vi "2DNonlinear Lev-Mar Fit.vi"(5 "Standard Deviation":dbl[](array[numeric]) format="%.2f", 7 "Function":refnum<vi>, 8 "max iteration":i32=200, 9 "Initial Guess Coefficients":dbl[](array[numeric]) format="%.2f", 10 "Y":dbl[](array[numeric]) format="%.2f", 11 "X":dbl[](array[numeric]) format="%.2f") -> (0 "error":i32, 1 "mse":dbl format="%.4e", 2 "Best Fit":dbl[](array[numeric]) format="%.2f", 3 "Best Fit Coefficients":dbl[](array[numeric]) format="%.2f", 4 "Covariance":dbl[][](array[numeric]) format="%.2f")   [LabVIEW 2016]
doc: "NonLinear Lev-Mar Fit:\n==================\n\nThis VI uses the Levenberg-Marquardt algorithm to determine the least squares set of coefficients that best fit the set of input data points(X,Y) as expressed by a nonlinear function y=f(x,a) where a is the set of coefficients. This VI also gives the best fit curve y=f(x.a). \n\nThe user needs to open a sub-VI \"Target Fnc & Deriv NonLin\" and inputs his/her nonlinear function f(x,a) in the Formula Node. If the user choose formula caculation for derivative method, he/she needs to input the partial deriative of f(x,a) with respect to a as well. \n\nInputs:\nX: experiment data points.\nY: experiment data points.\nStandard Deviation: standard deviation of each experiment data.If you don't have knowledge about this parameter, just leave it empty.\nInitial Guess Coefficients: Your guessed coefficients. If this is too far from the appropriate coefficients, the VI maybe will fail to return the appropriate coeficients and best fit curve.\nmax iteration: max iteration the algrothim will try. If it can not converge when it reaches the max iteration. The VI will return an error.\nderivative: There are two ways to caculate the partial derivative of f(x,a) with respect to coefficients a. If you choose nemerical caculation, the VI will use numerical method to caculate them internally. If you choose formula caculation, you need to input the derivative formula in the subvi Target Fnc & Deriv NonLin. formula caculation is more precise than numerical caculation.\n\nOutputs:\nBest Guess Coefficients: the least squares coefficients.\nBest Fit: the best fit curve f(x,a).\nCovariance: covariance matrix of Best Guess Coefficients.\nmse: mse=1/n*sum[(y(i)-f(x(i),a))/std(i)]^2)\n (std: Standard Deviation)"
uses:
  <vilib>/Analysis/baseanly.llb/Real Inverse Matrix.vi
  <vilib>/Analysis/NI_AALPro.lvlib
  <vilib>/Analysis/NI_AALBase.lvlib
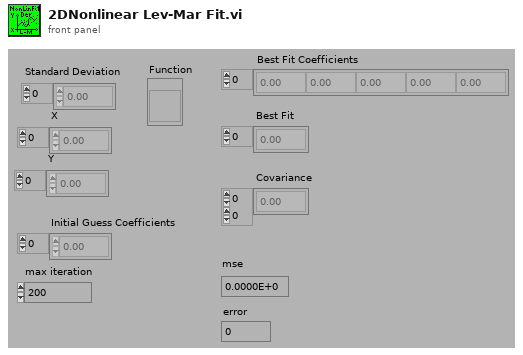
[diagram p1: front panel]
types:
  T1 = typedef "NI_Matrix.lvlib/RealMatrix.ctl" = dbl[][]
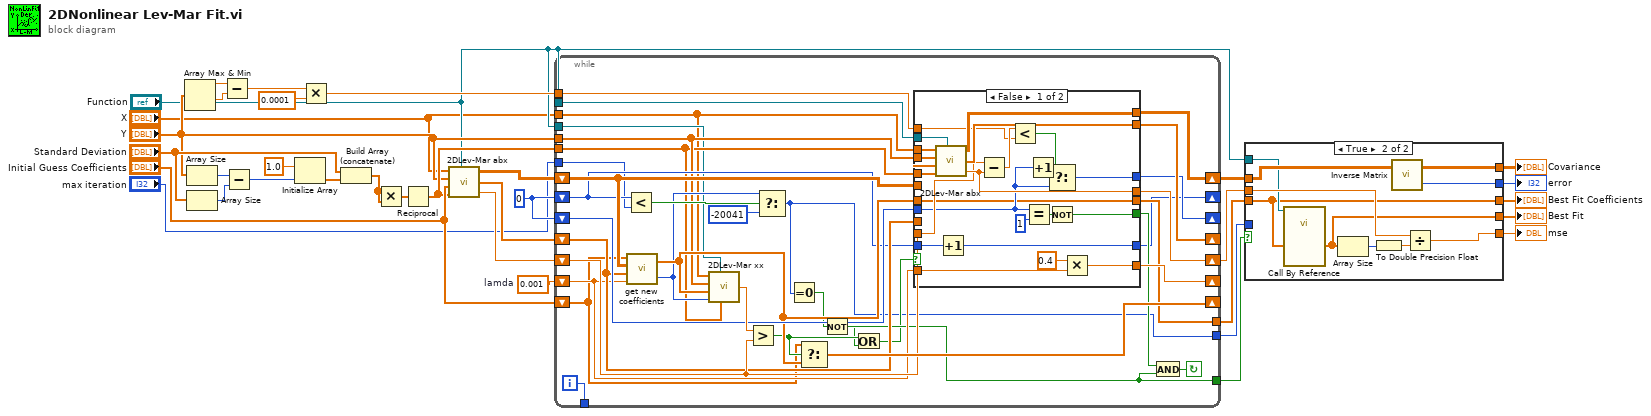
[diagram p0: block diagram]
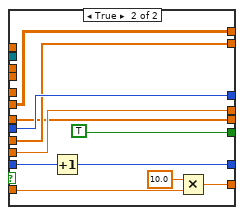
[diagram p2: hidden frame]
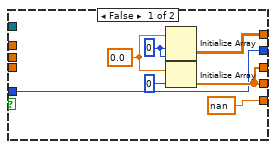
[diagram p3: hidden frame]
diagram:
  w25 = 0
  w33 = 0.001  # lamda
  n1 = Array Max & Min(array="Y") -> (max value=w7:dbl, min value=w6:dbl)  [unwired: 2 out]
  n2 = Array Size(array="Y") -> (size(s)=w13:i32)
  n3 = Array Size(array="Standard Deviation") -> (size(s)=w14:i32)
  n4 = Subtract(x=w7, y=w6) -> (x-y=w5:dbl)
  n5 = Subtract(x=w13, y=w14) -> (x-y=w15:i32)
  n6 = Initialize Array(1.0, w15) -> (w16:dbl[])
  n7 = Multiply(x=w5, y=0.0001) -> (x*y=w4:dbl)
  n8 = Build Array (concatenate)("Standard Deviation", w16) -> (w9:dbl[])
  n9 = Multiply(x=w9, y=w9) -> (x*y=w11:dbl[])
  n10 = Reciprocal(x=w11) -> (1/x=w10:dbl[])
  n11 = call "2DLev-Mar abx.vi"("X"="X", "Function"="Function", "Y"="Y", "Coefficients"="Initial Guess Coefficients", "W"=w10) -> ("Alpha"=w34:dbl[][], "Beta"=w32:dbl[], "chiSqr"=w31:dbl)  [unwired: 1 in]
  n12 = while {
    tunnel: "Function" -> [w37]
    tunnel: "Function" -> [w38]
    shift-right: [w68] -> _
    shift-left: w33 -> [w57]
    shift-right: [w67] -> _
    shift-left: "Initial Guess Coefficients" -> [w40]
    shift-right: [w66] -> w18
    shift-left: w34 -> [w65]
    shift-right: [w64] -> _
    shift-left: w32 -> [w59]
    shift-right: [w63] -> w30
    shift-left: w31 -> [w62]
    shift-right: [w60] -> _
    shift-left: w25 -> [w61]
    tunnel: [w56] -> w29
    tunnel: [w53] -> w26
    tunnel: w4 -> [w52]
    shift-right: [w48] -> _
    shift-left: w25 -> [w47]
    tunnel: "max iteration" -> [w43]
    tunnel: [w42] -> w19
    tunnel: "Y" -> [w41]
    tunnel: w10 -> [w39]
    tunnel: "X" -> [w36]
    tunnel: [w35] -> _
    i -> [w35]
    stop <- w55 continue-if-true
    n13 = Less?(x=w47, y=w43) -> (x < y?=w46:bool)
    n14 = call <vilib>:"get new coefficients.vi"("lamda"=w57, "Beta"=w59, "Alpha"=w65, "Coefficients"=w40) -> ("error"=w44:i32, "New Coefficients"=w58:dbl[])
    n15 = call "2DLev-Mar xx.vi"("W"=w39, "Function"=w37, "error"=w44, "Coefficients"=w58, "Y"=w41, "X"=w36) -> ("chiSqr"=w69:dbl)
    n16 = Greater?(x=w69, y=w62) -> (0:w50:bool)
    n17 = Select(t=w44, s=w46, f=-20041) -> (s? t:f=w42:i32)
    n18 = Equal To 0?(x=w42) -> (x = 0?=w53:bool)
    n19 = Select(t=w40, s=w50, f=w58) -> (s? t:f=w67:dbl[])
    n20 = Not(x=w53) -> (.not. x?=w49:bool)
    n21 = Or(x=w50, y=w49) -> (x .or. y?=w51:bool)
    n22 = case shown="False" w51 {
      tunnel: w57 -> [w91 w102]
      tunnel: [w90 w101] -> w68
      tunnel: [w89 w100] -> w66
      tunnel: w65 -> [_ w100]
      tunnel: [w88 w96] -> w64
      tunnel: [w87 w99] -> w63
      tunnel: w62 -> [w86 w99]
      tunnel: w61 -> [w81 w98]
      tunnel: [w82 w98] -> w60
      tunnel: [w78 TRUE] -> w54
      tunnel: w58 -> [w75 w95]
      tunnel: w59 -> [_ w96]
      tunnel: [w75 w95] -> w56
      tunnel: w52 -> [w77 _]
      tunnel: [w74 w94] -> w48
      tunnel: w47 -> [w76 w93]
      tunnel: w41 -> [w73 _]
      tunnel: w39 -> [w72 _]
      tunnel: w38 -> [w71 _]
      tunnel: w36 -> [w70 _]
      frame False {
        n23 = call "2DLev-Mar abx.vi"("X"=w70, "Function"=w71, "Y"=w73, "Coefficients"=w75, "W"=w72) -> ("Alpha"=w89:dbl[][], "Beta"=w88:dbl[], "chiSqr"=w87:dbl)  [unwired: 1 in]
        n24 = Increment(x=w76) -> (x+1=w74:i32)
        n25 = Subtract(x=w86, y=w87) -> (x-y=w85:dbl)
        n26 = Less?(x=w85, y=w77) -> (x < y?=w84:bool)
        n27 = Equal?(x=w81, y=1) -> (x = y?=w79:bool)
        n28 = Increment(x=w81) -> (x+1=w83:i32)
        n29 = Select(t=w83, s=w84, f=w81) -> (s? t:f=w82:i32)
        n30 = Not(x=w79) -> (.not. x?=w78:bool)
        n31 = Multiply(x=0.4, y=w91) -> (x*y=w90:dbl)
      }
      frame True {
        n32 = Increment(x=w93) -> (x+1=w94:i32)
        n33 = Multiply(x=10.0, y=w102) -> (x*y=w101:dbl)
      }
    }
    n34 = And(x=w54, y=w53) -> (x .and. y?=w55:bool)
  }
  n35 = case shown="True" w26 {
    tunnel: w29 -> [_ w113]
    tunnel: [w108 w113] -> w28
    tunnel: [nan w120] -> w27
    tunnel: [w108 w114] -> w22
    tunnel: w30 -> [_ w119]
    tunnel: [w106 w118] -> w21
    tunnel: [w105 w117] -> w20
    tunnel: w19 -> [w105 _]
    tunnel: w18 -> [_ w116]
    tunnel: "Function" -> [_ w115]
    frame False {
      w104 = 0.0 ("Element Data")
      w107 = 0
      n36 = Initialize Array(w104, w107, w107) -> (w106:dbl[][])
      n37 = Initialize Array(w104, 0) -> (w108:dbl[])
    }
    frame True {
      n38 = call-by-ref "?"(reference=w115, "Paramters"=w113) -> ("Simulated Image"=w114:dbl[])  [unwired: 1 in, 2 out]
      n39 = Array Size(array=w114) -> (size(s)=w112:i32)
      n40 = To Double Precision Float(number=w112) -> (double precision float=w111:dbl)
      n41 = call-poly <vilib>:"Inverse Matrix.vi"("Input Matrix"=w116) -> ("error"=w117:i32, "Inverse Matrix"=w118:T1)  [unwired: 1 in]
      n42 = Divide(x=w119, y=w111) -> (x/y=w120:dbl)
    }
  }
  "mse" <- w27
  "Best Fit Coefficients" <- w28
  "Best Fit" <- w22
  "error" <- w20
  "Covariance" <- w21
